vi "example.vi"() -> ()   [LabVIEW 2021]
uses:
  Users/olaja/AppData/Local/CETONI_SDK/lib/labview/labbCAN_Bus_API/SiUnitPrefix.ctl
  Users/olaja/AppData/Local/CETONI_SDK/lib/labview/labbCAN_Bus_API/TimeUnits.ctl
  Users/olaja/AppData/Local/CETONI_SDK/lib/labview/labbCAN_Pump_API/VolumeUnits.ctl
  CetoniPump.lvclass
  Users/olaja/AppData/Local/CETONI_SDK/lib/labview/labbCAN_Bus_API/labbCAN_Bus_API.lvlib
  Users/olaja/AppData/Local/CETONI_SDK/lib/labview/labbCAN_Pump_API/labbCAN_Pump_API.lvlib
panel:
  in  "SyringeSettings":T4={"Prefix"=-3, "TimeUnit"=60, "VolumeUnit"=68, "Maximum Piston Stroke (mm)"=100.0, "Inner Diameter (mm)"=12.0} {"VolumeUnit" items=["LITRES"=68]; "TimeUnit" items=["PER_SECOND"=1, "PER_MINUTE"=60, "PER_HOUR"=3600]; "Prefix" items=["UNIT"=0, "DECI"=-1, "CENTI"=-2, "MILLI"=-3, "MICRO"=-6]}
  in  "Cycle":bool
  in  "Flow Rate":dbl
  in  "Configure Syringe":bool
  out "Actual Flow Rate":dbl
  out "Is pumping":bool
  out "Fill Level":dbl
  in  "Level(ml)":dbl
  in  "Set Fill Level":bool
  in  "Generate FLow":bool
  in  "StopDosing":bool
  in  "Device Configuration Path":string="C:\\Users\\Public\\Documents\\QmixElements\\Projects\\default_project\\Configurations\\sinle"
  in  "Empty":bool
  in  "Refill":bool
  in  "Exit":bool
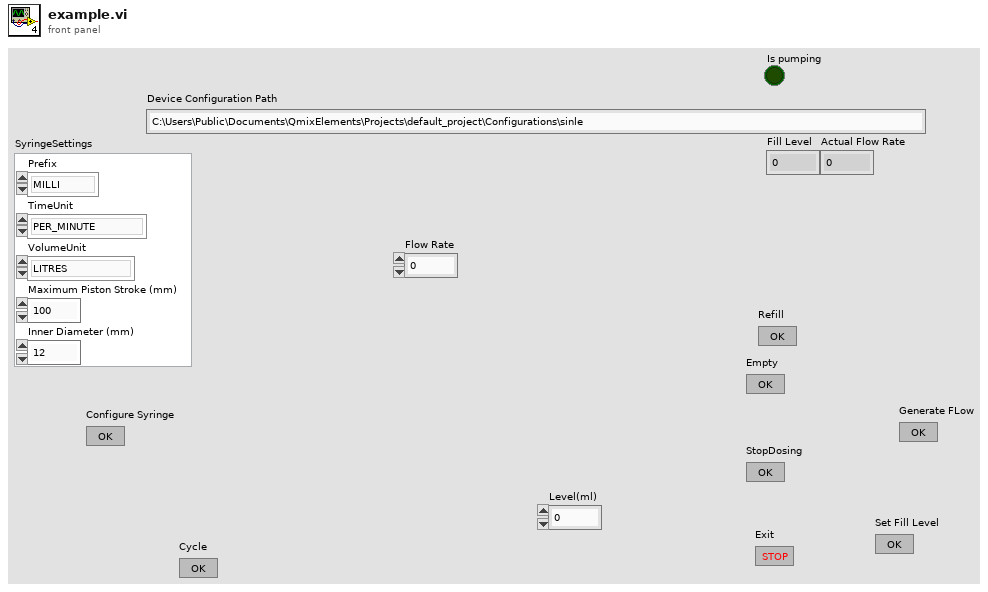
[diagram p1: front panel]
types:
  T1 = typedef "labbCAN_Bus_API.lvlib/SiUnitPrefix.ctl" = i32
  T2 = typedef "labbCAN_Bus_API.lvlib/TimeUnits.ctl" = i32
  T3 = typedef "labbCAN_Pump_API.lvlib/VolumeUnits.ctl" = i32
  T4 = cluster{"Prefix":T1, "TimeUnit":T2, "VolumeUnit":T3, "Maximum Piston Stroke (mm)":dbl, "Inner Diameter (mm)":dbl}
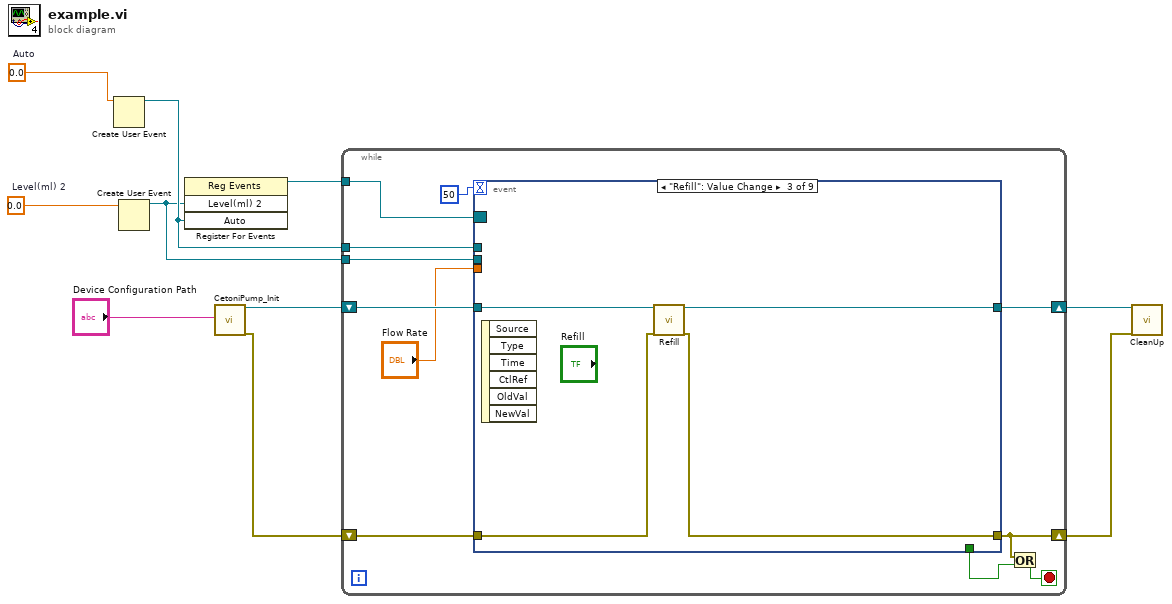
[diagram p0: block diagram]
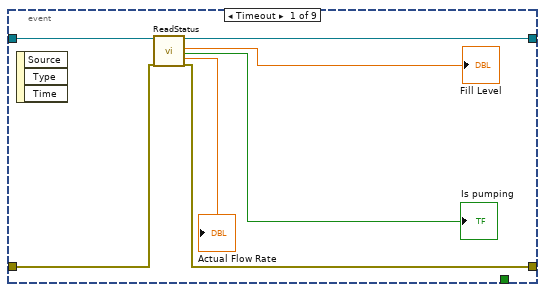
[diagram p2: hidden frame]
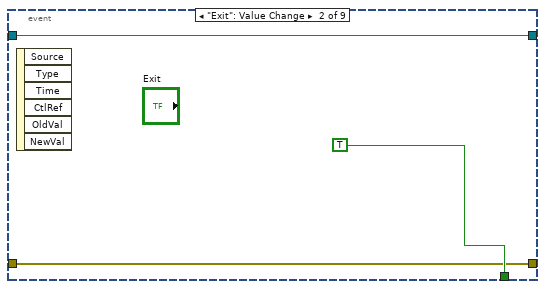
[diagram p3: hidden frame]
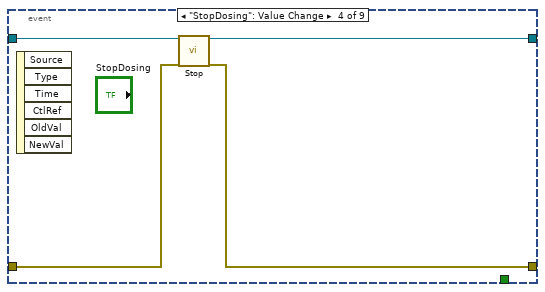
[diagram p4: hidden frame]
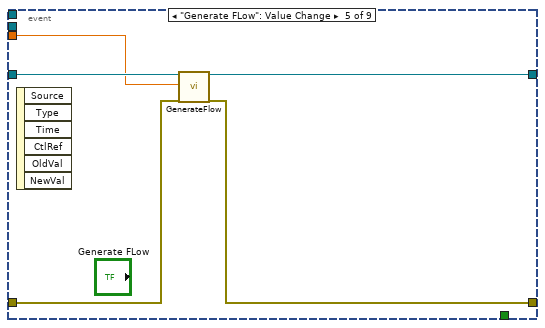
[diagram p5: hidden frame]
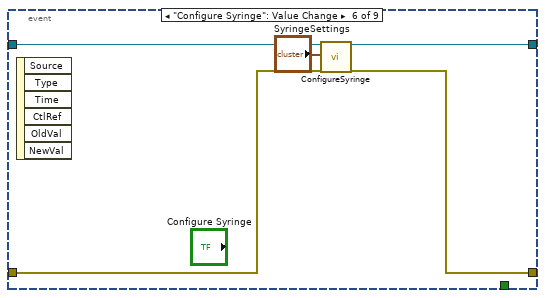
[diagram p6: hidden frame]
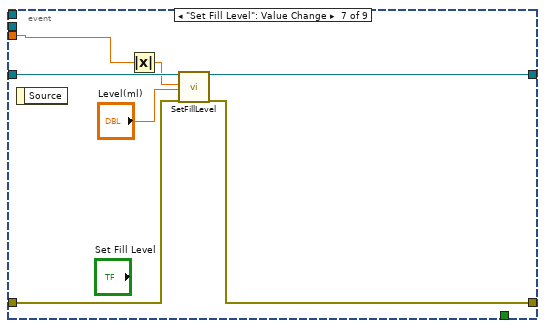
[diagram p7: hidden frame]
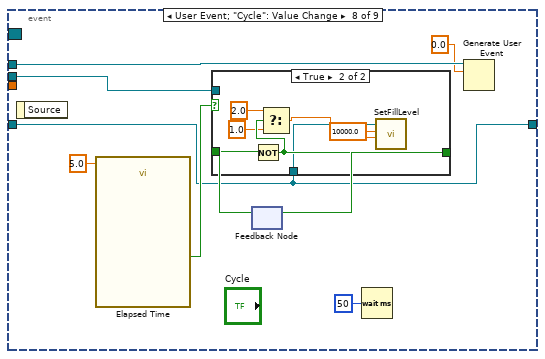
[diagram p8: hidden frame]
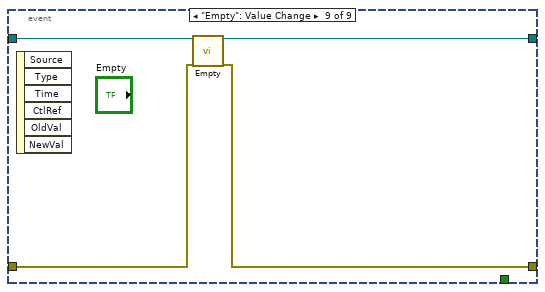
[diagram p10: hidden frame]
diagram:
  w3 = 0.0  # Auto
  w4 = 0.0  # Level(ml) 2
  n1 = Create User Event(user event datatype=w3) -> (user event=w2:refnum<user-event>)  [unwired: 1 in, 1 out]
  n2 = Create User Event(user event datatype=w4) -> (user event=w1:refnum<user-event>)  [unwired: 1 in, 1 out]
  n3 = register-events(w1, w2) -> (reference out=w5:refnum<event-registration>)  [unwired: 2 in, 1 out]
  n4 = call "CetoniPump_Init.vi"("Device Configuration Path"="Device Configuration Path") -> ("object out"=w10:refnum<class "CetoniPump.lvclass">, "error out"=w8:errorcluster)  [unwired: 17 in]
  n5 = while {
    shift-right: [w20] -> w9
    shift-left: w10 -> [w21]
    shift-right: [w18] -> w7
    shift-left: w8 -> [w19]
    tunnel: w5 -> [w13]
    tunnel: w2 -> [w12]
    tunnel: w1 -> [w11]
    stop <- w16 stop-if-true
    n6 = event shown="[2] \"Refill\": Value Change" {
      selector: w13 -> [_ _ _ _ _ _ _ _ _]
      dyn-events: _ -> [_ _ _ _ _ _ _ _ _]
      timeout: 50 -> [_ _ _ _ _ _ _ _ _]
      tunnel: w21 -> [w25 w30 w35 w38 w43 w48 w55 w58 w77]
      tunnel: [w26 w30 w34 w37 w42 w47 w54 w58 w76] -> w20
      tunnel: w19 -> [w28 w29 w33 w39 w44 w49 w56 _ w75]
      tunnel: [w27 w29 w32 w36 w41 w46 w53 _ w74] -> w18
      tunnel: [_ TRUE _ _ _ _ _ _ _] -> w17
      tunnel: "Flow Rate" -> [_ _ _ _ w40 _ w51 _ _]
      tunnel: w12 -> [_ _ _ _ _ _ _ w65 _]
      tunnel: w11 -> [_ _ _ _ _ _ _ w64 _]
      event Timeout {
        n7 = event-data() -> ()  [unwired: 1 in, 3 out]
        n8 = call-dynamic "ReadStatus.vi"("object in"=w25, "error in (no error)"=w28) -> ("object out"=w26:refnum<class "CetoniPump.lvclass">, "Fill Level"=→"Fill Level":dbl, "Is pumping"=→"Is pumping":bool, "Actual Flow Rate"=→"Actual Flow Rate":dbl, "error out"=w27:errorcluster)  [unwired: 13 in]
      }
      event "Exit": Value Change {
        n9 = event-data() -> ()  [unwired: 1 in, 6 out]
      }
      event "Refill": Value Change {
        n10 = event-data() -> ()  [unwired: 1 in, 6 out]
        n11 = call-dynamic "Refill.vi"("object in"=w35, "error in (no error)"=w33) -> ("object out"=w34:refnum<class "CetoniPump.lvclass">, "error out"=w32:errorcluster)  [unwired: 16 in]
      }
      event "StopDosing": Value Change {
        n12 = event-data() -> ()  [unwired: 1 in, 6 out]
        n13 = call-dynamic "Stop.vi"("object in"=w38, "error in (no error)"=w39) -> ("object out"=w37:refnum<class "CetoniPump.lvclass">, "error out"=w36:errorcluster)  [unwired: 16 in]
      }
      event "Generate FLow": Value Change {
        n14 = event-data() -> ()  [unwired: 1 in, 6 out]
        n15 = call-dynamic "GenerateFlow.vi"("object in"=w43, "Flow Rate"=w40, "error in (no error)"=w44) -> ("object out"=w42:refnum<class "CetoniPump.lvclass">, "error out"=w41:errorcluster)  [unwired: 15 in]
      }
      event "Configure Syringe": Value Change {
        n16 = event-data() -> ()  [unwired: 1 in, 6 out]
        n17 = call-dynamic "ConfigureSyringe.vi"("object in"=w48, "SyringeSettings"="SyringeSettings", "error in (no error)"=w49) -> ("object out"=w47:refnum<class "CetoniPump.lvclass">, "error out"=w46:errorcluster)  [unwired: 15 in]
      }
      event "Set Fill Level": Value Change {
        n18 = event-data() -> ()  [unwired: 1 in, 1 out]
        n19 = Absolute Value(x=w51) -> (abs(x)=w50:dbl)
        n20 = call-dynamic "SetFillLevel.vi"("object in"=w55, "Flow"=w50, "Level(ml)"="Level(ml)", "error in (no error)"=w56) -> ("object out"=w54:refnum<class "CetoniPump.lvclass">, "error out"=w53:errorcluster)  [unwired: 14 in]
      }
      event User Event; "Cycle": Value Change {
        n21 = event-data() -> ()  [unwired: 1 in, 1 out]
        n22 = call "Elapsed Time"("Time Target (s)"=5.0) -> ("Time has Elapsed"=w63:bool)  [unwired: 11 in, 7 out]
        n23 = feedback #1() -> (w62:bool)  [unwired: 1 in]
        n24 = case shown="True" w63 {
          tunnel: w64 -> [_ _]
          tunnel: w62 -> [w66 w73]
          tunnel: [w66 w72] -> w61
          tunnel: w58 -> [_ w69]
          frame False {
          }
          frame True {
            n25 = Not(x=w73) -> (.not. x?=w72:bool)
            n26 = Select(t=2.0, s=w72, f=1.0) -> (s? t:f=w67:dbl)
            n27 = call-dynamic "SetFillLevel.vi"("object in"=w69, "Flow"=10000.0, "Level(ml)"=w67) -> ()  [unwired: 15 in, 2 out]
          }
        }
        n28 = feedback-in #1(w61) -> ()
        n29 = Wait (ms)(milliseconds to wait=u32 50) -> ()  [unwired: 1 out]
        n30 = Generate User Event(user event=w65, event data cluster=0.0 ("event data")) -> ()  [unwired: 2 in, 2 out]
      }
      event "Empty": Value Change {
        n31 = event-data() -> ()  [unwired: 1 in, 6 out]
        n32 = call-dynamic "Empty.vi"("object in"=w77, "error in (no error)"=w75) -> ("object out"=w76:refnum<class "CetoniPump.lvclass">, "error out"=w74:errorcluster)  [unwired: 16 in]
      }
    }
    n33 = Or(x=w18, y=w17) -> (x .or. y?=w16:bool)
  }
  n34 = call-dynamic "CleanUp.vi"("object in"=w9, "error in (no error)"=w7) -> ()  [unwired: 16 in, 2 out]
